vi "Function.vi"(8 "error in (no error)":errorcluster, 10 "Numeric A":T1, 11 "Two Terminal in":refnum<class "AbsFunc_One Term_Complex SGL.lvclass">) -> (0 "error out":errorcluster, 2 "Result":T1, 3 "Two Terminal out":refnum<class "AbsFunc_One Term_Complex SGL.lvclass">)   [LabVIEW 2021, in "AbsFunc_One Term_Complex SGL.lvclass"]
uses:
  AbsFunc_One Term_Complex SGL.lvclass
  Support/Data Type.ctl
  AbsFunc_One Term_Complex SGL.lvclass/AbsFunc_One Term_Complex SGL.ctl
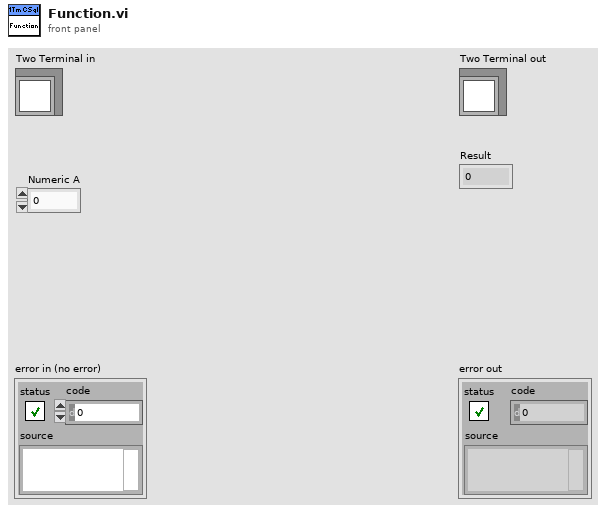
[diagram p1: front panel]
types:
  T1 = typedef "AbsFunc_One Term_Complex SGL.lvclass/Data Type.ctl" = csg
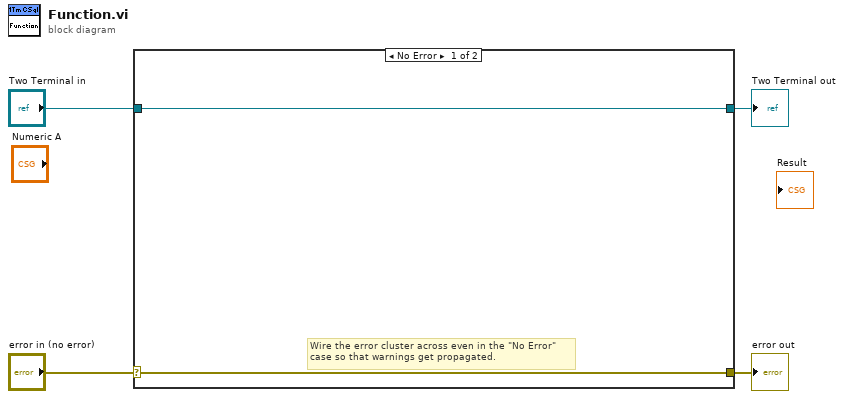
[diagram p0: block diagram]
diagram:
  n1 = case shown="No Error" "error in (no error)" {
    selector: "error in (no error)" -> [w5 w8]
    tunnel: [w5 w8] -> w3
    tunnel: [w6 w7] -> w1
    tunnel: "Two Terminal in" -> [w6 w7]
    frame No Error {
      # "Wire the error cluster across even in the \"No Error\"\ncase so that warnings get propagated."
    }
    frame Error {
    }
  }
  "error out" <- w3
  "Two Terminal out" <- w1
